vi "MB Modbus Demo Box Example.vi"() -> ()   [LabVIEW 2011]
uses:
  MB Serial Master Query Read Coils (poly).vi
  MB Serial Master Query Read Holding Registers (poly).vi
  MB Serial Master Query Write Multiple Coils (poly).vi
  MB Serial Master Query Write Multiple Registers (poly).vi
panel:
  in  "Ouputs":u16[](array[slide]) max=60 scale=0.0..60.0
  in  "Digital Outputs":T1
  out "Analog Inputs":T2 {"AI 5" scale=0.0..100.0; "AI 4" scale=0.0..100.0; "AI 3" scale=0.0..100.0; "AI 2" scale=0.0..100.0; "AI 1" scale=0.0..100.0}
  out "Digital Inputs":T3
  in  "COM Port":refnum<visa-resource-name>
  in  "Power":bool
  out "Power LED":bool
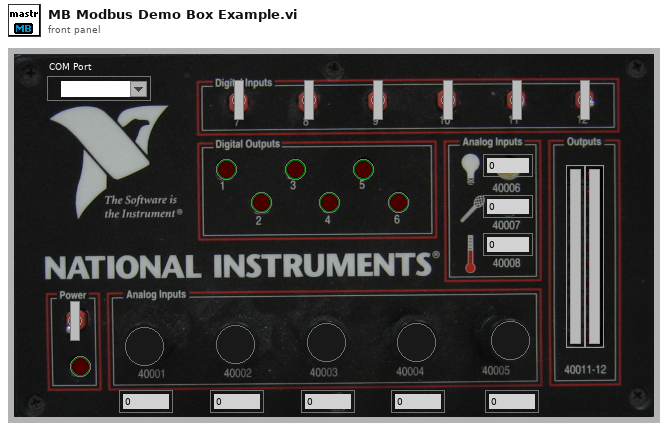
[diagram p1: front panel]
types:
  T1 = cluster{"DO 1":bool, "DO 2":bool, "DO 3":bool, "DO 4":bool, "DO 5":bool, "DO 6":bool}
  T2 = cluster{"AI 1":u16, "AI 2":u16, "AI 3":u16, "AI 4":u16, "AI 5":u16, "40006":u16, "40007":u16, "40008":u16}
  T3 = cluster{"DI1":bool, "DI1 2":bool, "DI1 3":bool, "DI1 4":bool, "DI1 5":bool, "DI1 6":bool}
  T4 = cluster{"Mode":enum16{"RTU", "ASCII"}, "Slave Address":u8}
  T5 = cluster{"Coils[0]":bool, "Coils[1]":bool, "Coils[2]":bool, "Coils[3]":bool, "Coils[4]":bool, "Coils[5]":bool}
  T6 = cluster{"Holding Registers[0]":u16, "Holding Registers[1]":u16, "Holding Registers[2]":u16, "Holding Registers[3]":u16, "Holding Registers[4]":u16, "Holding Registers[5]":u16, "Holding Registers[6]":u16, "Holding Registers[7]":u16}
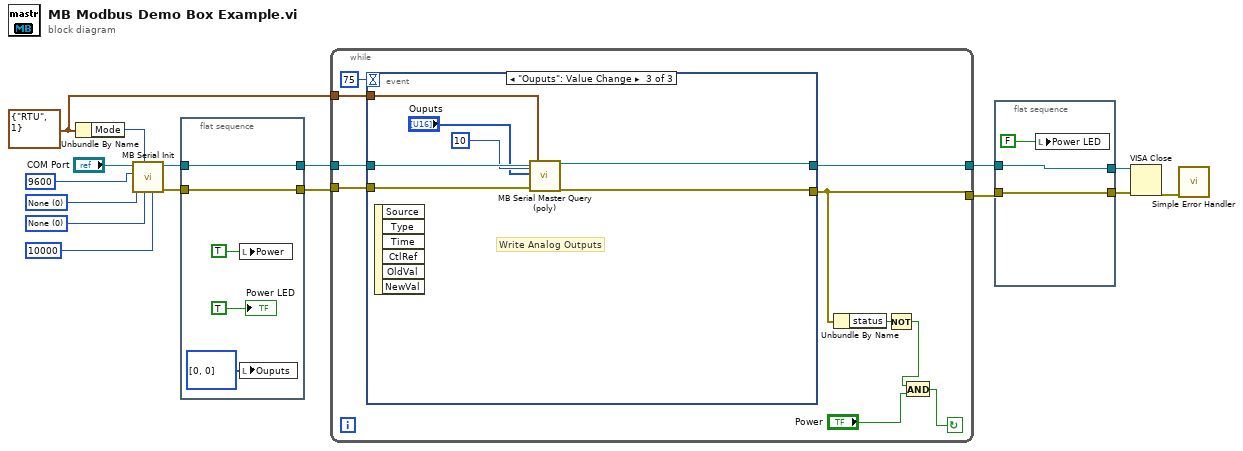
[diagram p0: block diagram]
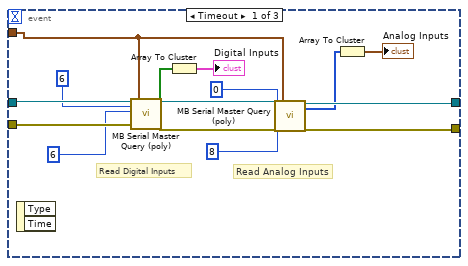
[diagram p2: hidden frame]
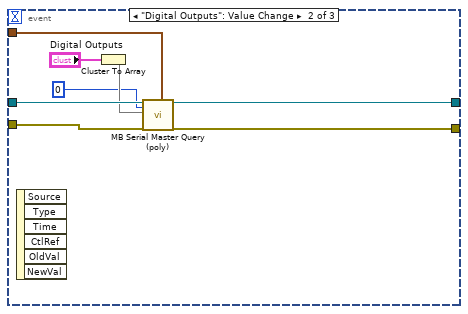
[diagram p3: hidden frame]
diagram:
  w6 = T4 {"Mode"=enum."RTU", "Slave Address"=1} ("Serial Parameters")
  w13 = u16 0 items=["None", "XON/XOFF", "RTS/CTS", "XON/XOFF & RTS/CTS", "DTR/DSR", "XON/XOFF & DTR/DSR"] ("Flow Control")
  w14 = u16 0 items=["None", "Odd", "Even", "Mark", "Space"] ("Parity")
  n1 = Unbundle By Name(w6) -> ("Mode"=w7:enum16{"RTU", "ASCII"})
  n2 = call "MB Serial Init.vi"("Timeout"=u32 10000, "Flow Control"=w13, "Mode"=w7, "Parity"=w14, "Baud Rate"=u32 9600, "VISA resource name"="COM Port") -> ("error out"=w10:errorcluster, "VISA resource name out"=w8:refnum<visa-resource-name>)  [unwired: 1 in, 3 out]
  n3 = flat-sequence {
    tunnel: [w18] -> w11
    tunnel: w10 -> [w18]
    tunnel: [w17] -> w9
    tunnel: w8 -> [w17]
    frame #0 {
      n4 = local write "Power"(TRUE ("Power")) -> ()
      n5 = local write "Ouputs"(u16[] [0, 0] ("Ouputs")) -> ()
      "Power LED" <- TRUE ("Power LED")
    }
  }
  n6 = while {
    tunnel: w9 -> [w31]
    tunnel: w11 -> [w29]
    tunnel: w6 -> [w30]
    tunnel: [w26] -> w5
    tunnel: [w25] -> w3
    stop <- w27 continue-if-true
    n7 = event shown="[2] \"Ouputs\": Value Change" {
      selector: _ -> [_ _ _]
      dyn-events: _ -> [_ _ _]
      timeout: 75 -> [_ _ _]
      tunnel: w31 -> [w46 w54 w61]
      tunnel: w30 -> [w36 w51 w60]
      tunnel: w29 -> [w45 w50 w59]
      tunnel: [w34 w48 w58] -> w25
      tunnel: [w35 w47 w57] -> w26
      event Timeout {
        # "Read Analog Inputs"
        # "Read Digital Inputs"
        n8 = event-data() -> ()  [unwired: 3 out]
        n9 = call-poly "MB Serial Master Query (poly).vi"("VISA resource name"=w46, "Starting Address"=u16 6, "Quantity"=u16 6, "error in"=w45, "Serial Parameters"=w36) -> ("VISA resource name out"=w40:refnum<visa-resource-name>, "Coils"=w41:bool[], "error out"=w39:errorcluster)  [unwired: 1 in, 11 out]
        n10 = Array To Cluster(array=w41) -> (cluster=→"Digital Inputs":T5)
        n11 = call-poly "MB Serial Master Query (poly).vi"("VISA resource name"=w40, "Starting Address"=u16 0, "Quantity"=u16 8, "error in"=w39, "Serial Parameters"=w36) -> ("VISA resource name out"=w35:refnum<visa-resource-name>, "Holding Registers"=w32:u16[], "error out"=w34:errorcluster)  [unwired: 1 in, 11 out]
        n12 = Array To Cluster(array=w32) -> (cluster=→"Analog Inputs":T6)
      }
      event "Digital Outputs": Value Change {
        n13 = event-data() -> ()  [unwired: 7 out]
        n14 = Cluster To Array(cluster="Digital Outputs") -> (array=w52:bool[])
        n15 = call-poly "MB Serial Master Query (poly).vi"("VISA resource name"=w54, "Starting Address"=u16 0, "Coils"=w52, "error in"=w50, "Serial Parameters"=w51) -> ("VISA resource name out"=w47:refnum<visa-resource-name>, "error out"=w48:errorcluster)  [unwired: 2 in, 11 out]
      }
      event "Ouputs": Value Change {
        # "Write Analog Outputs"
        n16 = event-data() -> ()  [unwired: 7 out]
        n17 = call-poly "MB Serial Master Query (poly).vi"("VISA resource name"=w61, "Starting Address"=u16 10, "Registers"="Ouputs", "error in"=w59, "Serial Parameters"=w60) -> ("VISA resource name out"=w57:refnum<visa-resource-name>, "error out"=w58:errorcluster)  [unwired: 2 in, 11 out]
      }
    }
    n18 = Unbundle By Name(w25) -> ("status"=w23:bool)
    n19 = Not(x=w23) -> (.not. x?=w22:bool)
    n20 = And(x=w22, y="Power") -> (x .and. y?=w27:bool)
  }
  n21 = flat-sequence {
    tunnel: w5 -> [w63]
    tunnel: [w63] -> w4
    tunnel: w3 -> [w62]
    tunnel: [w62] -> w2
    frame #0 {
      n22 = local write "Power LED"(FALSE ("Power LED")) -> ()
    }
  }
  n23 = VISA Close(VISA resource name=w4, error in (no error)=w2) -> (error out=w1:errorcluster)
  n24 = call <vilib>:"Simple Error Handler.vi"("error in (no error)"=w1) -> ()  [unwired: 1 in, 8 out]
